vi "CleanUp.vi"(11 "Python Code":string) -> (3 "spreadsheet string":string)   [LabVIEW 2020]
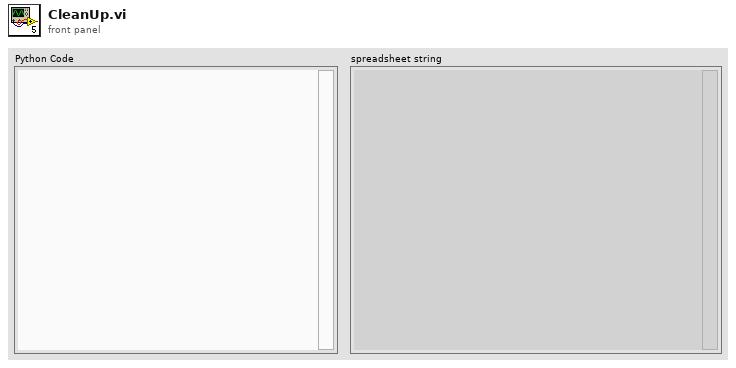
[diagram p1: front panel]
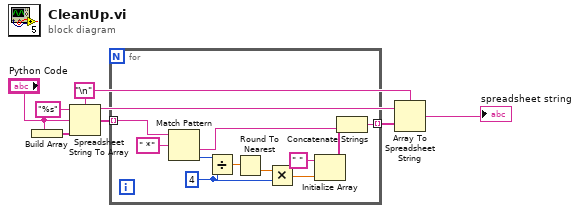
[diagram p0: block diagram]
diagram:
  w6 = "\n" ("delimiter (Tab)")
  w5 = "%s" ("format string")
  n1 = Build Array("Python Code") -> (w2:string[])
  n2 = Spreadsheet String To Array(delimiter (Tab)=w6, format string=w5, spreadsheet string="Python Code", array type (2D Dbl)=w2) -> (array=w3:string[])
  n3 = for {
    tunnel: w3 -> [w18] mode=indexing
    tunnel: [w8] -> w4 mode=indexing
    w13 = 4 ("y")
    n4 = Match Pattern(string=w18, regular expression=" *") -> (after substring=w9:string, offset past match=w16:i32)  [unwired: 1 in, 2 out]
    n5 = Divide(x=w16, y=w13) -> (x/y=w15:dbl)
    n6 = Round To Nearest(number=w15) -> (nearest integer value=w14:dbl)
    n7 = Multiply(x=w14, y=w13) -> (x*y=w12:dbl)
    n8 = Initialize Array(" " ("delimiter (Tab)"), w12) -> (w10:string[])
    n9 = Concatenate Strings(w10, w9) -> (w8:string)
  }
  n10 = Array To Spreadsheet String(delimiter (Tab)=w6, array=w4, 3:w5) -> (spreadsheet string=→"spreadsheet string":string)
